vi "SubEthernetSettings.vi"() -> (0 "Ethernet IP Address 2":string)   [LabVIEW 2020]
panel:
  in  "Cancel Button":bool
  in  "OK Button":bool
  in  "Ethernet IP Address":string="192.168.0.250"
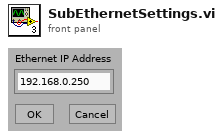
[diagram p1: front panel]
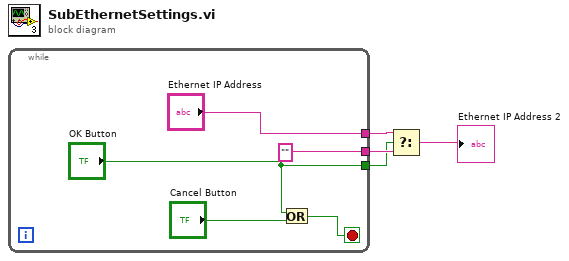
[diagram p0: block diagram]
diagram:
  n1 = while {
    tunnel: ["Ethernet IP Address"] -> w3
    tunnel: ["" ("f")] -> w2
    tunnel: ["OK Button"] -> w1
    stop <- w9 stop-if-true
    n2 = Or(x="OK Button", y="Cancel Button") -> (x .or. y?=w9:bool)
  }
  n3 = Select(t=w3, s=w1, f=w2) -> (s? t:f=→"Ethernet IP Address 2":string)
